vi "PDF T90.vi"(8 "error in (no error)":errorcluster caption="Fehler (Eingang, kein Fehler)", 10 "SVGraph Referenz":refnum<vi>, 11 "seconds since 1Jan1904":timestamp) -> (0 "error out":errorcluster caption="Fehler (Ausgang)")   [LabVIEW 2020, in "T90.lvlib"]
uses:
  T90.lvlib
  Schedule Modul/Aktion FGV Testdaten sammeln.ctl
  Sprachverwaltung/FGV Aktion Tabelle zerlegen.ctl
  Linearisierung V2/Protokoll/Protokoll.lvlib
  Schedule Modul/Schedule Modul.lvlib
  Sprachverwaltung/Sprachverwaltung.lvlib
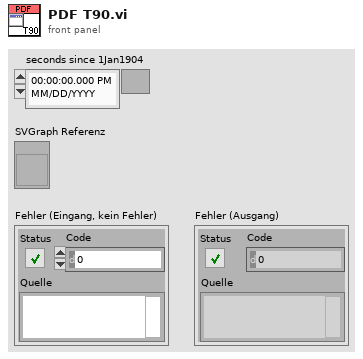
[diagram p1: front panel]
types:
  T1 = typedef "Sprachverwaltung.lvlib/FGV Aktion Tabelle zerlegen.ctl" = enum16{"laden", "vereinzeln", "speichern"}
  T2 = typedef "Schedule Modul.lvlib/Aktion FGV Testdaten sammeln.ctl" = enum16{"lesen", "Dichtheitstest", "CalGasTest", "T90", "Kalibrieren", "init", "Kalender Daten"}
  T3 = typedef "Schedule Modul.lvlib/Ergebnis T90.ctl" = cluster{"T90":waveform(sgl), "T10:":T4, "T50:":T4, "T90:":T4, "Rise Time":T4, "Leitungslänge":T5, "Fehler":bool}
  T4 = typedef "Zahlen-Ausgabefeld.ctl" = sgl
  T5 = typedef "Zahlen-Eingabefeld.ctl" = sgl
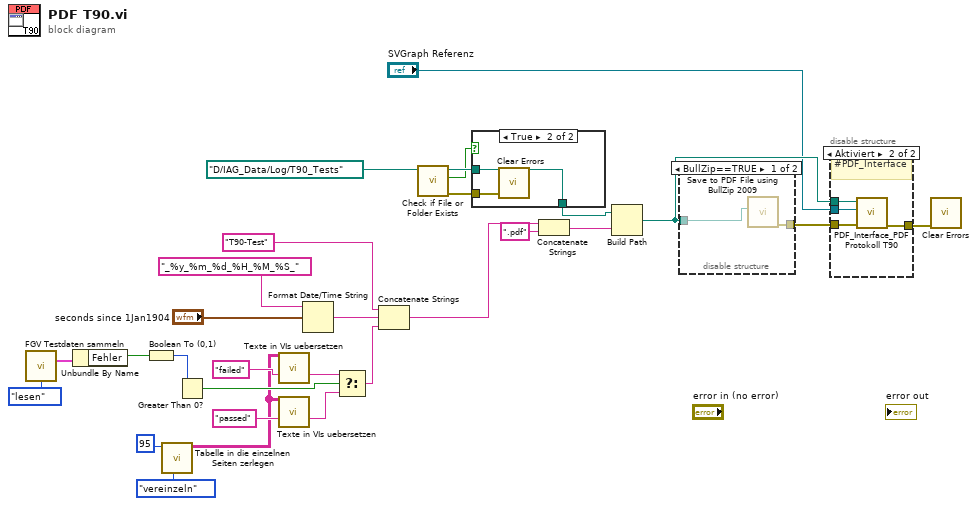
[diagram p0: block diagram]
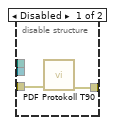
[diagram p2: hidden frame]
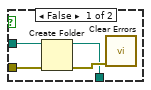
[diagram p3: hidden frame]
diagram:
  n1 = call "FGV Testdaten sammeln.vi"("Aktion"=Aktion_FGV_Testdaten_sammeln."lesen") -> ("Ergebnis T90"=w16:T3)  [unwired: 9 in, 5 out]
  n2 = Unbundle By Name(w16) -> ("Fehler"=w14:bool)
  n3 = Boolean To (0,1)(Boolean=w14) -> (0, 1=w15:i16)
  n4 = call "Tabelle in die einzelnen Seiten zerlegen.vi"("Aktion"=FGV_Aktion_Tabelle_zerlegen."vereinzeln", "Index (Seite)"=95) -> ("Sprachliste"=w3:string[][])  [unwired: 7 in, 2 out]
  n5 = Greater Than 0?(x=w15) -> (x > 0?=w4:bool)
  n6 = call "Texte in VIs uebersetzen.vi"("Sprachliste"=w3, "String zum Übersetzen"="failed" ("String")) -> ("String zum Übersetzen"=w7:string)  [unwired: 9 in, 4 out]
  n7 = call "Texte in VIs uebersetzen.vi"("Sprachliste"=w3, "String zum Übersetzen"="passed" ("String")) -> ("String zum Übersetzen"=w6:string)  [unwired: 9 in, 4 out]
  n8 = Format Date/Time String(time format string (%c)="_%y_%m_%d_%H_%M_%S_" ("Zeitformatierungs-String (%c)"), seconds (now)="seconds since 1Jan1904") -> (date/time string=w22:string)  [unwired: 1 in]
  n9 = Select(t=w7, s=w4, f=w6) -> (s? t:f=w5:string)
  n10 = Concatenate Strings("T90-Test" ("String"), w22, w5) -> (w24:string)
  n11 = call <vilib>:"Check if File or Folder Exists.vi"("path"=path "D:/IAG_Data/Log/T90_Tests" ("Pfad:")) -> ("error out"=w29:errorcluster, "file or folder exists?"=w26:bool, "dup path"=w27:path)  [unwired: 8 in]
  n12 = case shown="True" w26 {
    tunnel: w27 -> [w33 w35]
    tunnel: [w31 w35] -> w28
    tunnel: w29 -> [w30 w34]
    frame False {
      n13 = Create Folder(path (use dialog)=w33, error in=w30) -> (created path=w31:path, error out=w32:errorcluster)  [unwired: 1 in, 1 out]
      n14 = call <vilib>:"Clear Errors.vi"("error in (no error)"=w32) -> ()  [unwired: 5 in, 2 out]
    }
    frame True {
      n15 = call <vilib>:"Clear Errors.vi"("error in (no error)"=w34) -> ()  [unwired: 5 in, 2 out]
    }
  }
  n16 = Concatenate Strings(w24, ".pdf" ("String")) -> (w19:string)
  n17 = Build Path(base path=w28, name or relative path=w19) -> (appended path=w2:path)
  n18 = disable-structure shown="BullZip==TRUE" {
    disable-tunnel: [w37 _] -> w13
    disable-tunnel: w2 -> [w36 _]
    frame condition #0 {
      n19 = call "Save to PDF File using BullZip 2009.vi"("Save PDF File Path"=w36) -> ("error out"=w37:errorcluster)  [unwired: 10 in]
    }
    frame condition #1 (active) {
    }
  }
  n20 = disable-structure shown="Aktiviert" {
    disable-tunnel: w13 -> [w39 w43]
    disable-tunnel: [w38 w42] -> w12
    disable-tunnel: w2 -> [_ w41]
    disable-tunnel: "SVGraph Referenz" -> [_ w40]
    frame Disabled {
      n21 = call "PDF Protokoll T90.vi"("error in (no error)"=w39) -> ("error out"=w38:errorcluster)  [unwired: 10 in]
    }
    frame Enabled {
      # "#PDF_Interface"
      n22 = call "PDF_Interface_PDF Protokoll T90.vi"("error in (no error)"=w43, "SVGraph Referenz"=w40, "Save PDF File Path"=w41) -> ("error out"=w42:errorcluster)  [unwired: 8 in]
    }
  }
  n23 = call <vilib>:"Clear Errors.vi"("error in (no error)"=w12) -> ()  [unwired: 5 in, 2 out]
